vi "MotorControlTest.vi"() -> ()   [LabVIEW 2019, in "CubeMarsBLDClib.lvlib"]
uses:
  MotorParameters.ctl
  <vilib>/Platform/TimedLoop/XDataNode/timing_clust.ctl
  <vilib>/Platform/TimedLoop/XDataNode/nitl_modes.ctl
  <vilib>/Platform/TimedLoop/XDataNode/wakeup.ctl
  MotorType.ctl
  <vilib>/myRIO/Common/Instrument Driver Framework/myRIO v1.0/UART/vis/myRIO v1.0 Close UART.vi
  <vilib>/myRIO/Common/Instrument Driver Framework/Utilities/vis/FPGA Ref Manager.vi
  <vilib>/myRIO/Common/Instrument Driver Framework/myRIO v1.0/myRIO v1.0 Reset FPGA.vi
  <vilib>/myRIO/Common/Instrument Driver Framework/myRIO v1.0/IRQ/vis/myRIO v1.0 IRQ Info FGV.vi
  <vilib>/myRIO/Common/Instrument Driver Framework/myRIO v1.0/IRQ/vis/myRIO v1.0 Timer IRQ Info FGV.vi
  <vilib>/myRIO/Common/Instrument Driver Framework/myRIO v1.0/IRQ/vis/myRIO v1.0 ISR Agent.vi
  <vilib>/myRIO/Instrument Drivers/Utilities/vis/Reset Index.vi
  <vilib>/myRIO/Common/Instrument Driver Framework/myRIO v1.0/Resource Manager/vis/myRIO v1.0 Block Write Resource Manager.vi
  <vilib>/platform/TimedLoop/XDataNode/XDataNode.xnode
  CubeMarsBLDClib.lvlib
  <vilib>/myRIO/Instrument Drivers/Utilities/Utilities.lvlib
  <vilib>/Platform/TimedLoop/XDataNode/XDNodeRunTimeDep.lvlib
panel:
  out "FilteredValue":T1
  out "dt(ms)":dbl
  in  "Disable Motor":bool
  in  "ValueIn":T1
  in  "Enable Motor":bool
  out "error out":errorcluster
  in  "stop":bool
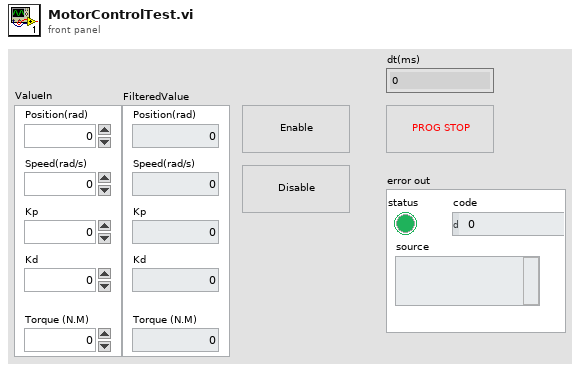
[diagram p1: front panel]
types:
  T1 = typedef "CubeMarsBLDClib.lvlib/MotorParameters.ctl" = cluster{"Position(rad)":dbl, "Speed(rad/s)":dbl, "Kp":dbl, "Kd":dbl, "Torque (N.M)":dbl}
  T2 = typedef "CubeMarsBLDClib.lvlib/MotorType.ctl" = enum16{"AK80-64"}
  T3 = typedef "CubeMarsBLDClib.lvlib/Reference.ctl" = cluster{"VISA resource name":refnum<visa-resource-name>, "MotorType":T2, "CAN ID":u32}
  T4 = typedef "XDNodeRunTimeDep.lvlib/timing_clust.ctl" = cluster{"Expected End [f-1]":u64, "Actual End [f-1]":u64, "Finished Late? [f-1]":bool, "Expected End [i-1]":u64, "Actual End [i-1]":u64, "Finished Late? [i-1]":bool, "Expected Start [i]":u64, "Actual Start [i]":u64, "Expected Start [f]":u64, "Actual Start [f]":u64, "Source Name":string, "Structure Name":string, "Period":i64, "Deadline":i64, "Offset":i64, "Start":i64, "Priority":i32, "Timeout":i32, "Mode":T5, "Wakeup Reason":T6, "Error":errorcluster, "Source Type":string, "Secondary Source Type":string, "Global End Time":u64, "Global Start Time":u64, "Frame Duration":u64, "Iteration Duration":u64, "Assigned CPU":i32, "I/O Scan Engine Mode":u32}
  T5 = typedef "XDNodeRunTimeDep.lvlib/nitl_modes.ctl" = enum32{"No Change", "Process missed periods, maintain original phase", "Discard missed periods, maintain original phase", "Process missed periods, ignore original phase", "Discard missed periods, ignore original phase"}
  T6 = typedef "XDNodeRunTimeDep.lvlib/wakeup.ctl" = enum32{"Normal", "Aborted", "Asynchronous wakeup", "Timing source error", "Timed loop error", "Timeout"}
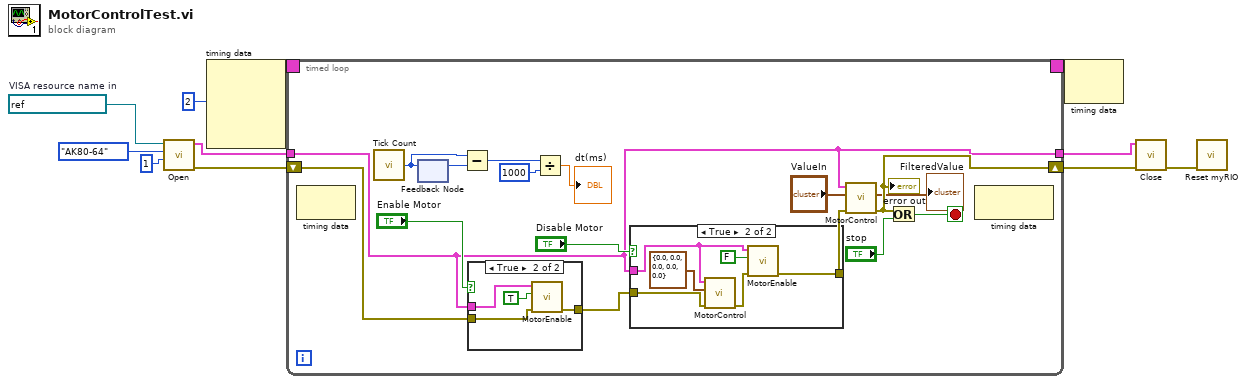
[diagram p0: block diagram]
diagram:
  w8 = refnum<visa-resource-name> "ASRL3::INSTR"  # VISA resource name in
  n1 = call "Open.vi"("CAN ID"=u32 1, "MotorType"=MotorType."AK80-64", "USB CAN VISA resource name"=w8) -> ("Error Out"=w4:errorcluster, "Reference Out"=w5:T3)  [unwired: 7 in]
  n2 = node-c288(i64 2 ("Period")) -> (w11:T4)  [unwired: 3 in]
  n3 = timed-loop {
    shift-right: [w22] -> w3
    shift-left: w4 -> [w27]
    timing: w11 -> [_]
    timing-out: [_] -> w10
    tunnel: w5 -> [w18]
    tunnel: [w18] -> w1
    stop <- w23 stop-if-true
    n4 = node-c288() -> ()  [unwired: 1 in, 1 out]
    n5 = call "Tick Count"() -> ("Tick Count(uSec)"=w17:u32)
    n6 = feedback-in #1(w17) -> ()
    n7 = feedback #1() -> (w16:u32)  [unwired: 1 in]
    n8 = Subtract(x=w17, y=w16) -> (x-y=w15:u32)
    n9 = case shown="True" "Enable Motor" {
      tunnel: w27 -> [w37 w41]
      tunnel: [w37 w40] -> w20
      tunnel: w18 -> [_ w39]
      frame False {
      }
      frame True {
        n10 = call "MotorEnable.vi"("Error In"=w41, "Enable?"=TRUE, "Reference In"=w39) -> ("Error Out"=w40:errorcluster)  [unwired: 7 in, 1 out]
      }
    }
    n11 = Divide(x=w15, y=u32 1000) -> (x/y=→"dt(ms)":dbl)
    n12 = case shown="True" "Disable Motor" {
      tunnel: w20 -> [w28 w32]
      tunnel: [w28 w33] -> w19
      tunnel: w18 -> [_ w30]
      frame False {
      }
      frame True {
        n13 = call "MotorControl.vi"("error in"=w32, "ValueIn"=T1 {"Position(rad)"=0.0, "Speed(rad/s)"=0.0, "Kp"=0.0, "Kd"=0.0, "Torque (N.M)"=0.0}, "Reference In"=w30) -> ("error out"=w31:errorcluster)  [unwired: 6 in, 2 out]
        n14 = call "MotorEnable.vi"("Error In"=w31, "Enable?"=FALSE, "Reference In"=w30) -> ("Error Out"=w33:errorcluster)  [unwired: 7 in, 1 out]
      }
    }
    n15 = call "MotorControl.vi"("error in"=w19, "ValueIn"="ValueIn", "Reference In"=w18) -> ("error out"=w22:errorcluster, "FilteredValue"=→"FilteredValue":T1)  [unwired: 6 in, 1 out]
    "error out" <- w22
    n16 = Or(x=w22, y="stop") -> (x .or. y?=w23:bool)
    n17 = node-c288() -> ()  [unwired: 1 in, 1 out]
  }
  n18 = node-c288(w10) -> ()  [unwired: 1 out]
  n19 = call "Close.vi"("Error In"=w3, "Reference IN"=w1) -> ("Error Out"=w2:errorcluster)  [unwired: 9 in]
  n20 = call <vilib>:"Reset myRIO.vi"("error in (no error)"=w2) -> ()  [unwired: 10 in, 1 out]
